vi "BloqueDeFormula.vi"() -> ()   [LabVIEW 2021]
panel:
  out "Numeric D":dbl
  out "Numeric C":dbl
  in  "Numeric B":dbl
  in  "Numeric A":dbl
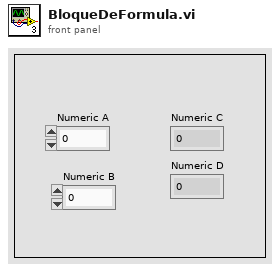
[diagram p1: front panel]
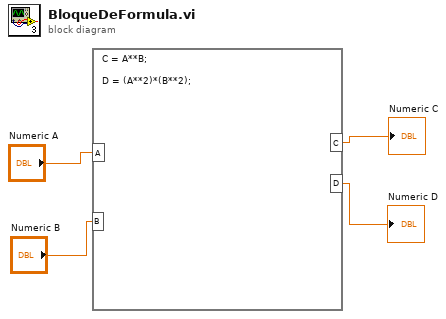
[diagram p0: block diagram]
diagram:
  n1 = formula code="C = A**B;\n\nD = (A**2)*(B**2);"("A"="Numeric A", "B"="Numeric B") -> ("C"=→"Numeric C":dbl, "D"=→"Numeric D":dbl)
